vi "Cam-color4.vi"(7 "error in":errorcluster) -> (20 "Classifier Session (Color Classification 1)":T2, 21 "Classes (Color Classification 1)":string[](array[string]), 27 "error out":errorcluster)   [LabVIEW 2018]
uses:
  <vilib>/vision/Classification.llb/IMAQ Classifier Session.ctl
  <vilib>/userdefined/High Color/IMAQdx.ctl
  <vilib>/vision/Classification.llb/IMAQ Classifier Read Options.ctl
  <vilib>/vision/NI_Vision_Development_Module.lvlib
  <vilib>/vision/driver/NI_Vision_Acquisition_Software.lvlib
panel:
  in  "error in 2":errorcluster
  out "Image Out":T1(plugin-control)
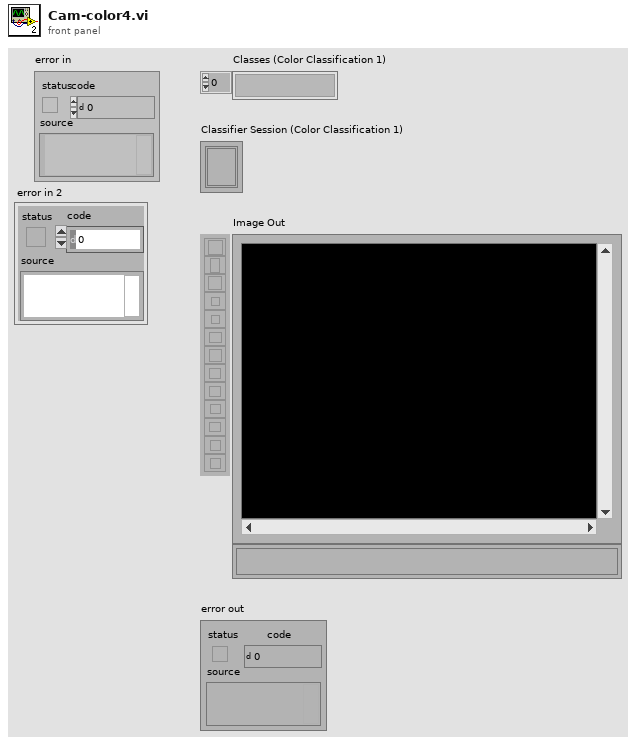
[diagram p1: front panel]
types:
  T1 = typedef "IMAQ Image.ctl" = refnum<image>
  T2 = typedef "IMAQ Classifier Session.ctl" = refnum<k1>
  T3 = typedef "IMAQdx.ctl" = refnum<k21>
  T4 = cluster{"Global Rectangle":i32[], "Contours":cluster{"ID":enum32{"External", "Internal"}, "Type":u32, "Coordinates":i32[]}[]}
  T5 = typedef "IMAQ Classifier Read Options.ctl" = i32
  T6 = typedef "ROI Descriptor" = cluster{"Global Rectangle":i32[], "Contours":cluster{"ID":enum32{"External", "Internal"}, "Type":u32, "Coordinates":i32[]}[]}
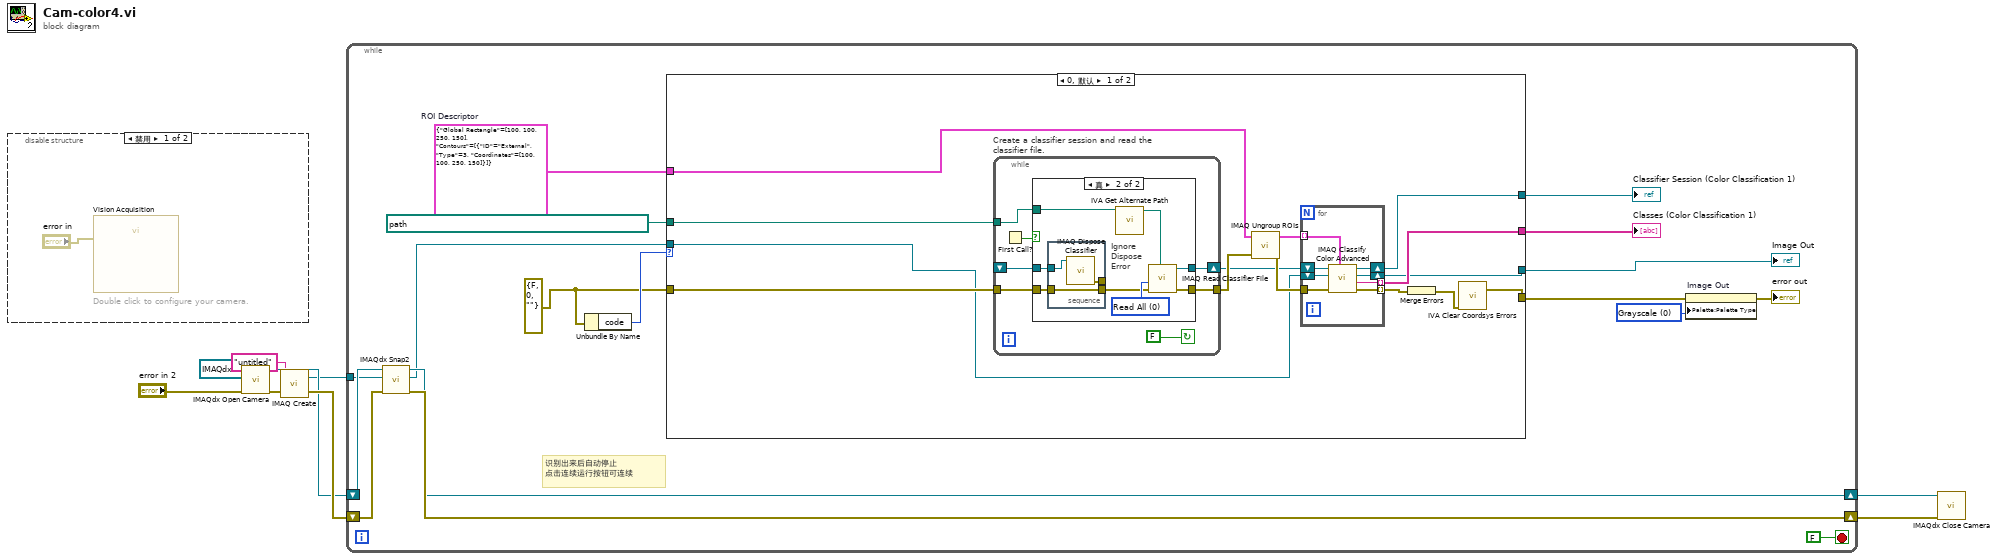
[diagram p0: block diagram]
diagram:
  n1 = disable-structure shown="禁用" {
    frame Disabled {
      # "Double click to configure your camera."
      n2 = call "Vision Acquisition"("error in"="error in") -> ()  [unwired: 25 in, 2 out]
    }
    frame Enabled {
    }
  }
  n3 = call <vilib>:"IMAQdx Open Camera.vi"("error in"="error in 2", "Session In"=T3 "cam1") -> ("error out"=w9:errorcluster, "Session Out"=w6:T3)  [unwired: 8 in]
  n4 = call "IMAQ Create"("Image Name"="untitled", "error in (no error)"=w9) -> ("New Image"=w4:T1, "error out"=w8:errorcluster)  [unwired: 3 in]
  n5 = while {
    tunnel: w4 -> [w16]
    shift-right: [w19] -> w7
    shift-left: w8 -> [w20]
    shift-right: [w17] -> w5
    shift-left: w6 -> [w18]
    stop <- FALSE stop-if-true
    w12 = errorcluster {"status"=FALSE, "code"=0, "source"=""} ("error out")
    w21 = u32 0 items=["Grayscale", "Binary", "Gradient", "Rainbow", "Temperature", "User Defined", "Binary 16 Bit", "Gradient 16 Bit", "Rainbow 16 Bit", "Temperature 16 Bit", "User Defined 16 Bit"] ("Palette Type")
    w26 = T4 {"Global Rectangle"=[100, 100, 250, 150], "Contours"=[{"ID"=enum."External", "Type"=3, "Coordinates"=[100, 100, 250, 150]}]}  # ROI Descriptor
    # "识别出来后自动停止\n点击连续运行按钮可连续"
    n6 = call <vilib>:"IMAQdx Snap2.vi"("error in"=w20, "Image In"=w16, "Session In"=w18) -> ("error out"=w19:errorcluster, "Image Out"=w15:T1, "Session Out"=w17:T3)  [unwired: 6 in]
    n7 = Unbundle By Name(w12) -> ("code"=w13:i32)
    n8 = case shown="0, 默认" w13 {
      tunnel: [w41 _] -> w27
      tunnel: w26 -> [w40 _]
      tunnel: [w34 _] -> w25
      tunnel: [w32 _] -> w24
      tunnel: [w31 _] -> w22
      tunnel: w12 -> [w30 _]
      tunnel: w15 -> [w29 _]
      tunnel: path "D:/Labviewprogram/视觉/视觉框架/Color 识别.clf" ("File Path") -> [w28 _]
      frame 0, Default {
        n9 = while "Create a classifier session and read the classifier file." {
          shift-right: [w56] -> w33
          shift-left: _ -> [w55]
          tunnel: w30 -> [w53]
          tunnel: [w52] -> w39
          tunnel: w28 -> [w50]
          stop <- FALSE continue-if-true
          n10 = First Call?() -> (First Call?: T/F=w51:bool)
          n11 = case "条件结构" shown="真" w51 {
            tunnel: [w58 w65] -> w56
            tunnel: w55 -> [w58 w63]
            tunnel: w53 -> [w57 w62]
            tunnel: [w57 w64] -> w52
            tunnel: w50 -> [_ w60]
            frame False {
            }
            frame True {
              w66 = T5 0 items=["Read All", "Add Samples, Do Not Change Options", "Read Options, Do Not Add Samples"] ("Read Options")
              # "Ignore Dispose Error"
              n12 = stacked-sequence "层叠式顺序结构" {
                tunnel: w63 -> [w69]
                tunnel: w62 -> [w68]
                tunnel: [w68] -> w61
                tunnel: [w67] -> _
                frame #0 {
                  n13 = call "IMAQ Dispose Classifier"("Classifier Session"=w69) -> ("error out"=w67:errorcluster)  [unwired: 1 in, 9 out]
                }
              }
              n14 = call <vilib>:"IVA Get Alternate Path.vi"("Path In"=w60) -> ("Path Out"=w59:path)  [unwired: 10 out]
              n15 = call "IMAQ Read Classifier File"("File Path"=w59, "error in (no error)"=w61, "Read Options"=w66) -> ("error out"=w64:errorcluster, "Classifier Session"=w65:T2)  [unwired: 1 in, 6 out]
            }
          }
        }
        n16 = call "IMAQ Ungroup ROIs"("error in (no error)"=w39, "ROI Descriptor"=w40) -> ("error out"=w38:errorcluster, "ROI Descriptors out"=w37:T6[])  [unwired: 2 out]
        n17 = for "For循环" {
          tunnel: [w49] -> w41 mode=indexing
          tunnel: [w48] -> w36 mode=indexing
          tunnel: w38 -> [w46]
          tunnel: w37 -> [w45] mode=indexing
          shift-right: [w43] -> w31
          shift-left: w29 -> [w44]
          shift-right: [w42] -> w32
          shift-left: w33 -> [w47]
          n18 = call "IMAQ Classify Color Advanced"("ROI Descriptor"=w45, "error in (no error)"=w46, "Image"=w44, "Classifier Session"=w47) -> ("error out"=w48:errorcluster, "Class"=w49:string, "Image (dup)"=w43:T1, "Classifier Session (dup)"=w42:T2)  [unwired: 4 out]
        }
        n19 = Merge Errors(w36) -> (w35:errorcluster)
        n20 = call <vilib>:"IVA Clear Coordsys Errors.vi"("error in (no error)"=w35) -> ("error out"=w34:errorcluster)  [unwired: 10 in]
      }
      frame 1 {
      }
    }
    "Classes (Color Classification 1)" <- w27
    "Classifier Session (Color Classification 1)" <- w24
    "Image Out" <- w22
    n21 = property on="Image Out" class="ImageControl"(error in=w25, "Palette:Palette Type"=w21) -> (error out=→"error out":errorcluster)  [unwired: 1 in, 1 out]
  }
  n22 = call <vilib>:"IMAQdx Close Camera.vi"("error in"=w7, "Session In"=w5) -> ()  [unwired: 9 in, 1 out]
